vi "Default global.vi"() -> ()   [LabVIEW 2014]
doc: "This global VI can contain as many global variables as you need. Place a control on the panel, give it a good name. To read or write to it from a VI, drag the icon to the diagram of that VI. You can also drag from the project. Click on the node to change which global you access. You shouldn't have multiple locations writing to a global or it will cause a race-condition."
uses:
  <vilib>/Rock Robotics/WPI/Camera/WPI_CameraImageSize.ctl
  <vilib>/Rock Robotics/WPI/DriverStation/WPI_DriverStationRobotMode2.ctl
panel:
  out "Base path":path
  out "Operator Controller":T1
  out "Driver controller":T1
  in  "Robot Mode":T2
  in  "image size":T3=enum."320x240"
  in  "Enable Vision":bool
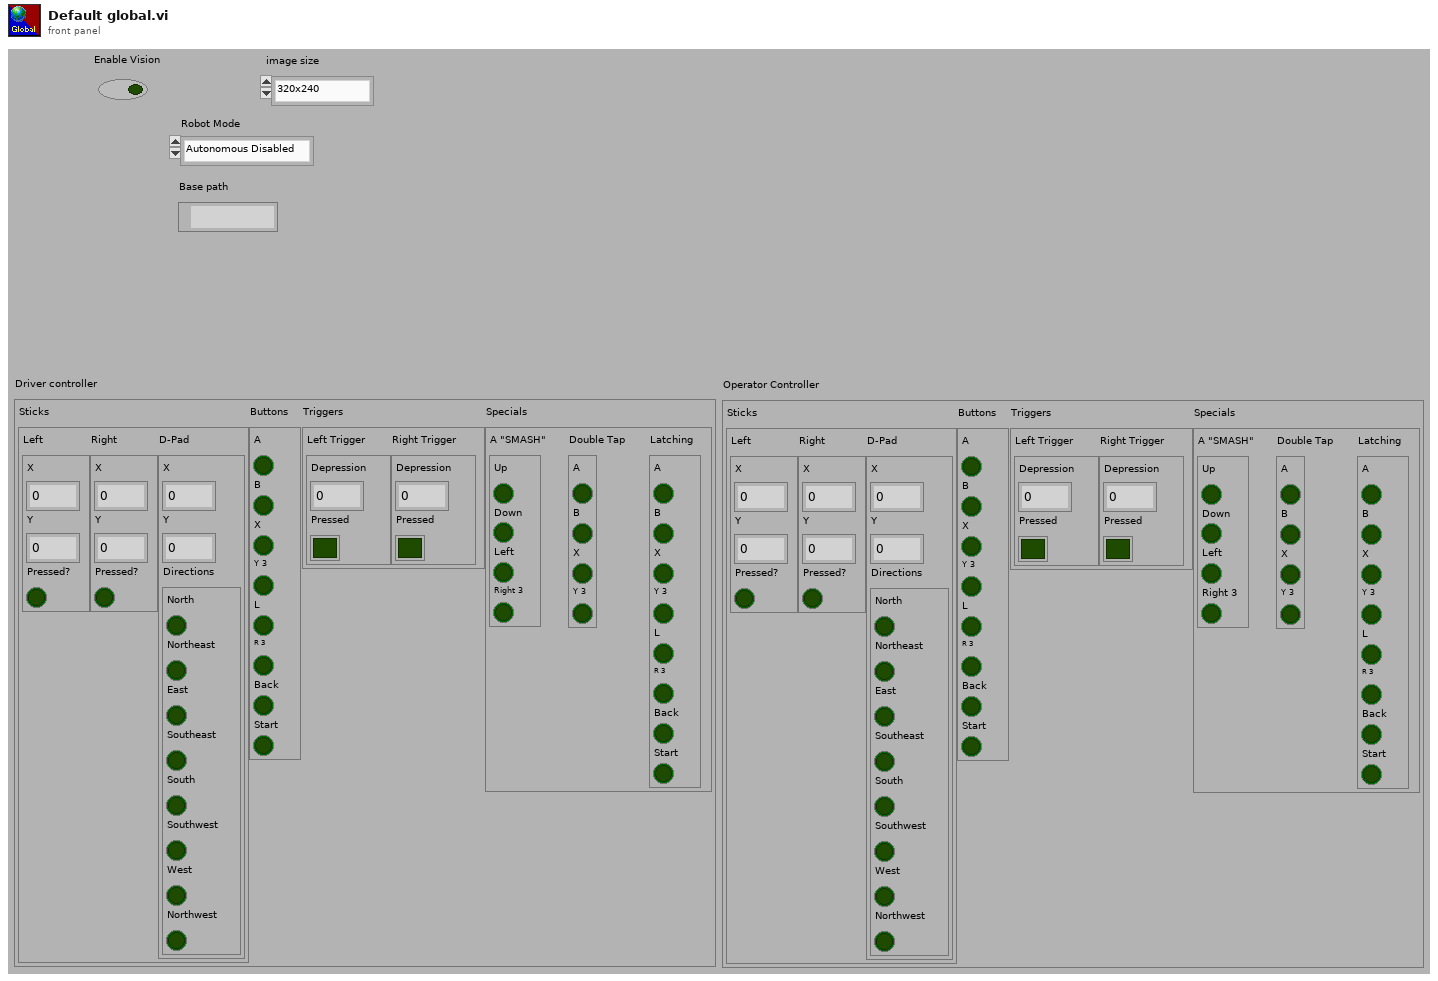
[diagram p1: front panel]
types:
  T1 = cluster{"Sticks":cluster{"Left":cluster{"X":dbl, "Y":dbl, "Pressed?":bool}, "Right":cluster{"X":dbl, "Y":dbl, "Pressed?":bool}, "D-Pad":cluster{"X":dbl, "Y":dbl, "Directions":cluster{"North":bool, "Northeast":bool, "East":bool, "Southeast":bool, "South":bool, "Southwest":bool, "West":bool, "Northwest":bool}}}, "Buttons":cluster{"A":bool, "B":bool, "X":bool, "Y 3":bool, "L":bool, "R 3":bool, "Back":bool, "Start":bool}, "Triggers":cluster{"Left Trigger":cluster{"Depression":dbl, "Pressed":bool}, "Right Trigger":cluster{"Depression":dbl, "Pressed":bool}}, "Specials":cluster{"A \"SMASH\"":cluster{"Up":bool, "Down":bool, "Left":bool, "Right 3":bool}, "Double Tap":cluster{"A":bool, "B":bool, "X":bool, "Y 3":bool}, "Latching":cluster{"A":bool, "B":bool, "X":bool, "Y 3":bool, "L":bool, "R 3":bool, "Back":bool, "Start":bool}}}
  T2 = typedef "WPI_DriverStationRobotMode2.ctl" = enum16{"Autonomous Disabled", "Autonomous Enabled", "Teleop Disabled", "Teleop Enabled", "Disconnected", "Finish", "Test Disabled", "Test Enabled", "Emergency Stopped"}
  T3 = typedef "WPI_CameraImageSize.ctl" = enum16{"640x480", "320x240", "160x120", "Custom"}
diagram:
